vi "Parse Header.vi"(10 "Header":string, 11 "XML in":refnum<class "XML.lvclass">) -> (1 "Value":string[](array[string]), 2 "Name":string[](array[string]), 3 "XML out":refnum<class "XML.lvclass">)   [LabVIEW 2019, in "XML.lvlib" / "XML.lvclass"]
uses:
  <vilib>/gpm_packages/@cs/persistence/source/XML/XML.lvclass
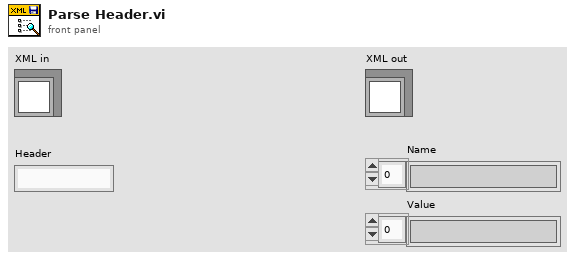
[diagram p1: front panel]
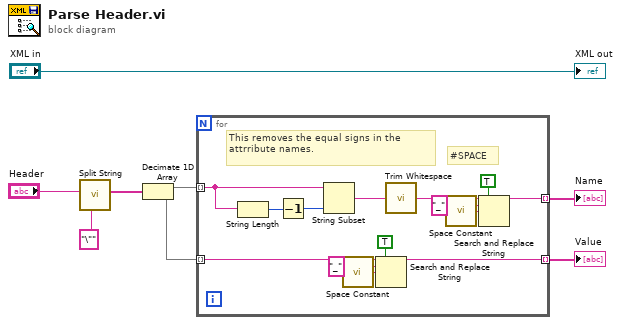
[diagram p0: block diagram]
diagram:
  n1 = call <vilib>:"Split String.vi"("Split Pattern"="\"", "Input String"="Header") -> ("Split String"=w5:string[])  [unwired: 9 in]
  n2 = Decimate 1D Array(w5) -> (w4:string[], w2:string[])
  n3 = for {
    tunnel: w4 -> [w21] mode=indexing
    tunnel: [w14] -> w3 mode=indexing
    tunnel: w2 -> [w10] mode=indexing
    tunnel: [w9] -> w1 mode=indexing
    # "#SPACE"
    # "This removes the equal signs in the\nattrribute names."
    n4 = String Length(string=w21) -> (length=w20:i32)
    n5 = Decrement(x=w20) -> (x-1=w19:i32)
    n6 = String Subset(string=w21, length (rest)=w19) -> (substring=w22:string)  [unwired: 1 in]
    n7 = call <vilib>:"Space Constant.vi"() -> ("String"=w13:string)
    n8 = Search and Replace String(replace all?=TRUE ("replace all? (F)"), input string=w10, search string="_" ("input string"), replace string=w13) -> (result string=w9:string)  [unwired: 4 in, 3 out]
    n9 = call <vilib>:"Trim Whitespace.vi"("string"=w22) -> ("trimmed string"=w15:string)  [unwired: 1 in]
    n10 = call <vilib>:"Space Constant.vi"() -> ("String"=w16:string)
    n11 = Search and Replace String(replace all?=TRUE ("replace all? (F)"), input string=w15, search string="_" ("input string"), replace string=w16) -> (result string=w14:string)  [unwired: 4 in, 3 out]
  }
  "Name" <- w3
  "Value" <- w1
  "XML out" <- "XML in"
